vi "readAttributes.vi"(8 "Fehler (Eingang, kein Fehler)":errorcluster, 10 "index":i32, 11 "Refnum in":refnum<k20>) -> (0 "Fehler (Ausgang)":errorcluster, 2 "size(s)":i32, 3 "Node Value 2":string)   [LabVIEW 2013, in "XML.lvlib"]
uses:
  lib/XML.lvlib
  <resource>/objmgr/DOMUserDefRef.rc
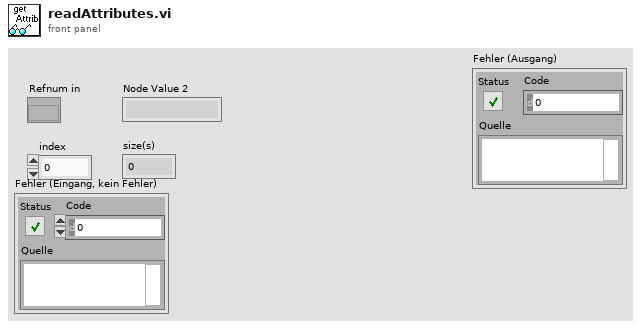
[diagram p1: front panel]
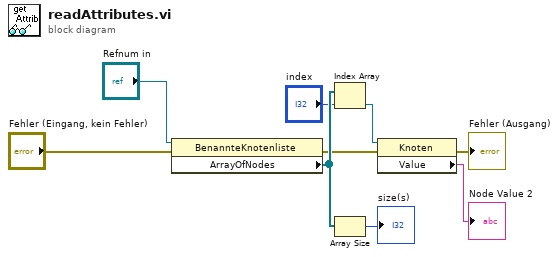
[diagram p0: block diagram]
diagram:
  n1 = property class="BenannteKnotenliste"(reference="Refnum in", error in="Fehler (Eingang, kein Fehler)") -> (error out=w3:errorcluster, "ArrayOfNodes"=w8:refnum<k20>[])  [unwired: 1 out]
  n2 = Index Array(array=w8, index="index") -> (element=w9:refnum<k20>)
  n3 = Array Size(array=w8) -> (size(s)=→"size(s)":i32)
  n4 = property class="Knoten"(reference=w9, error in=w3) -> (error out=→"Fehler (Ausgang)":errorcluster, "Value"=→"Node Value 2":string)  [unwired: 1 out]
